vi "Initialized Edit Sensor.vi"(8 "error in (no error)":errorcluster, 11 "Edit Sensor Model in":refnum<class "Edit Sensor Model.lvclass">) -> (0 "error out":errorcluster, 3 "Edit Sensor Model out":refnum<class "Edit Sensor Model.lvclass">)   [LabVIEW 2013, in "Edit Sensor Model.lvlib" / "Edit Sensor Model.lvclass"]
uses:
  Edit Sensor Model.lvclass
  Edit Sensor Model.lvclass/Edit Sensor Model.ctl
  <vilib>/ActorFrameworkMVC/View Observer/View Registry/View Registry.lvclass/View Registry.ctl
  Edit Sensor Model Messages/Abstract Initialize Edit Sensor Msg/Abstract Initialize Edit Sensor Msg.lvclass
  <vilib>/ActorFrameworkMVC/View Observer/Data Message/Data Message.lvclass
  <vilib>/ActorFrameworkMVC/View Observer/View Registry/View Registry.lvclass
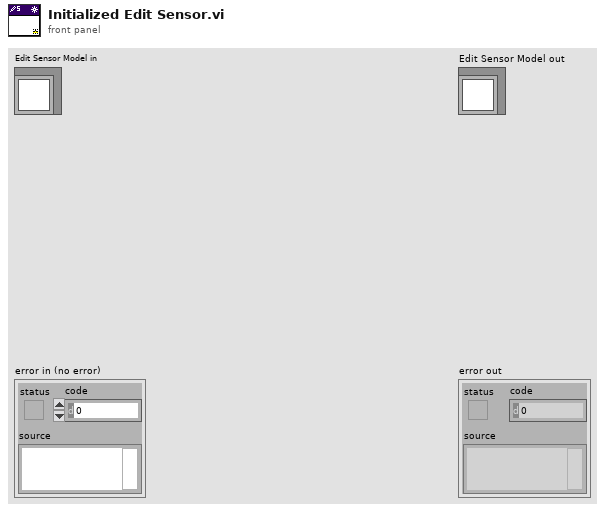
[diagram p1: front panel]
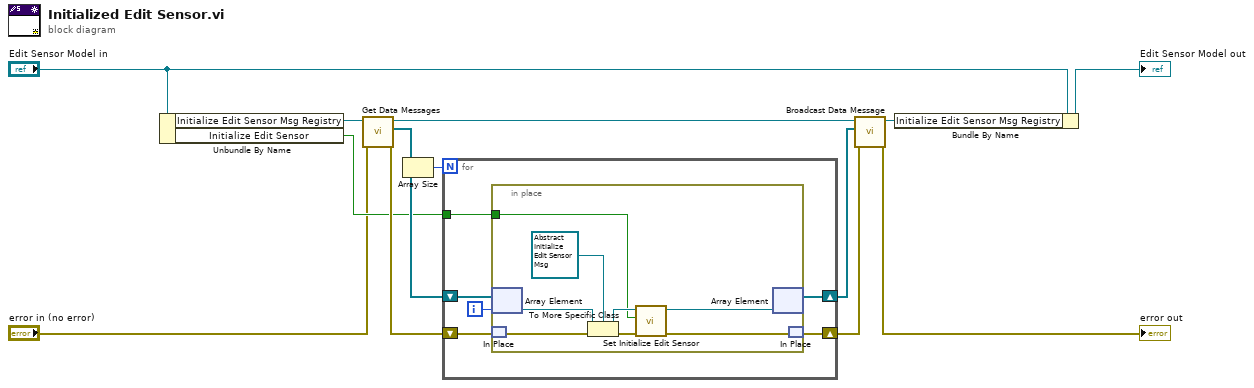
[diagram p0: block diagram]
diagram:
  n1 = Unbundle By Name("Edit Sensor Model in") -> ("Initialize Edit Sensor Msg Registry"=w13:refnum<class "View Registry.lvclass">, "Initialize Edit Sensor"=w8:bool)
  n2 = call <vilib>:"Get Data Messages.vi"("error in (no error)"="error in (no error)", "View Registry in"=w13) -> ("error out"=w9:errorcluster, "Data Messages"=w10:refnum<class "Data Message.lvclass">[], "View Registry out"=w12:refnum<class "View Registry.lvclass">)  [unwired: 7 in]
  n3 = Array Size(array=w10) -> (size(s)=w11:i32)
  n4 = for {
    N: w11 -> [_]
    shift-right: [w18] -> w7
    shift-left: w10 -> [w19]
    shift-right: [w15] -> w6
    shift-left: w9 -> [w17]
    tunnel: w8 -> [w16]
    i -> [w14]
    n5 = in-place {
      in-place-border: w16 -> [w20]
      n6 = in-place-array #1(w19, w14) -> (w25:refnum<class "Data Message.lvclass">)
      n7 = in-place-match #2(w17) -> (w27:errorcluster)
      n8 = To More Specific Class(target class=refnum<class "Abstract Initialize Edit Sensor Msg.lvclass"> refnum ("Edit Sensor Model.lvlib:Abstract Initialize Edit Sensor Msg.lvclass"), reference=w25, error in=w27) -> (specific class reference=w21:refnum<class "Abstract Initialize Edit Sensor Msg.lvclass">, error out=w24:errorcluster)
      n9 = call "Set Initialize Edit Sensor.vi"("error in (no error)"=w24, "Initialize Edit Sensor"=w20, "Abstract Initialize Edit Sensor Msg in"=w21) -> ("error out"=w23:errorcluster, "Abstract Initialize Edit Sensor Msg out"=w22:refnum<class "Abstract Initialize Edit Sensor Msg.lvclass">)  [unwired: 7 in]
      n10 = in-place-array #1(w22) -> (w18:refnum<class "Data Message.lvclass">[])  [unwired: 1 out]
      n11 = in-place-match #2(w23) -> (w15:errorcluster)
    }
  }
  n12 = call <vilib>:"Broadcast Data Message.vi"("error in (no error)"=w6, "Data Messages"=w7, "View Registry in"=w12) -> ("error out"=→"error out":errorcluster, "View Registry out"=w5:refnum<class "View Registry.lvclass">)  [unwired: 7 in]
  n13 = Bundle By Name(cluster="Edit Sensor Model in", "Initialize Edit Sensor Msg Registry"=w5) -> (→"Edit Sensor Model out":refnum<class "Edit Sensor Model.lvclass">)
